vi "Send Listening Queue.vi"(8 "error in (no error)":errorcluster, 11 "Generic Controller In":refnum<class "Generic Plugin.lvclass">) -> (0 "error out":errorcluster, 3 "Generic Controller Out":refnum<class "Generic Plugin.lvclass">)   [LabVIEW 2020, in "RxnRover.lvlib" / "Generic Plugin.lvclass"]
uses:
  Generic Plugin.lvclass
  Generic Plugin.lvclass/Generic Plugin.ctl
  <userlib>/RxnRover/DynamicReentrant/Dynamic Reentrant.lvlib
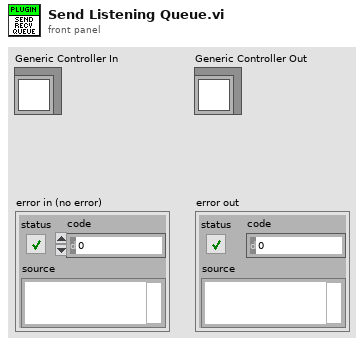
[diagram p1: front panel]
types:
  T1 = typedef "Dynamic Reentrant.lvlib/Message.ctl" = cluster{"Source":string, "Destination":string, "Time Stamp":timestamp, "Command":string, "Data":variant}
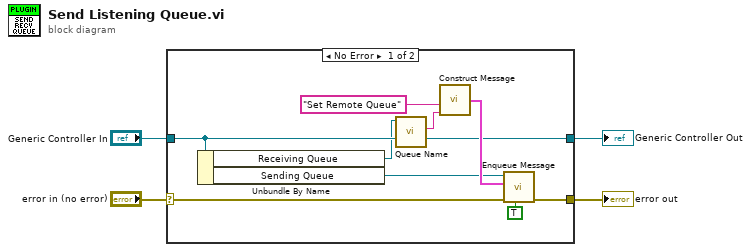
[diagram p0: block diagram]
diagram:
  n1 = case shown="No Error" "error in (no error)" {
    selector: "error in (no error)" -> [w7 w15]
    tunnel: [w10 w15] -> w4
    tunnel: "Generic Controller In" -> [w8 w14]
    tunnel: [w8 w14] -> w2
    frame No Error {
      n2 = Unbundle By Name(w8) -> ("Receiving Queue"=w6:refnum<queue>, "Sending Queue"=w9:refnum<queue>)
      n3 = call <userlib>:"Queue Name.vi"("Remote VI Queue in"=w6) -> ("Queue Name"=w5:string)  [unwired: 9 in, 1 out]
      n4 = call <userlib>:"Construct Message.vi"("Data"=w5, "Command"="Set Remote Queue") -> ("Message Cluster"=w12:T1)  [unwired: 4 in]
      n5 = call <userlib>:"Enqueue Message.vi"("Priority Message? (F)"=TRUE, "error in (no error)"=w7, "Message"=w12, "Listening Queue"=w9) -> ("error out"=w10:errorcluster)  [unwired: 6 in, 1 out]
    }
    frame Error {
    }
  }
  "error out" <- w4
  "Generic Controller Out" <- w2
